vi "Keithley Source Control Panel.vi"(8 "error in (no error)":errorcluster, 11 "Class":refnum<class "Keithley Source.lvclass">) -> (0 "error out":errorcluster, 3 "Keithley Source out":refnum<class "Keithley Source.lvclass">)   [LabVIEW 2015, in "Keithley Source.lvclass"]
uses:
  Keithley Source.lvclass
  Kethley Source Data.ctl
panel:
  in  "Data":T1={"Mode"=enum."up-down sweep", "Start current"=-2e-08, "End current"=2e-08, "Current step"=1e-09, "Compliance"=0.0} {"Compliance" format="%#_4p"; "Current step" format="%#_4p"; "End current" format="%#_4p"; "Start current" format="%#_4p"}
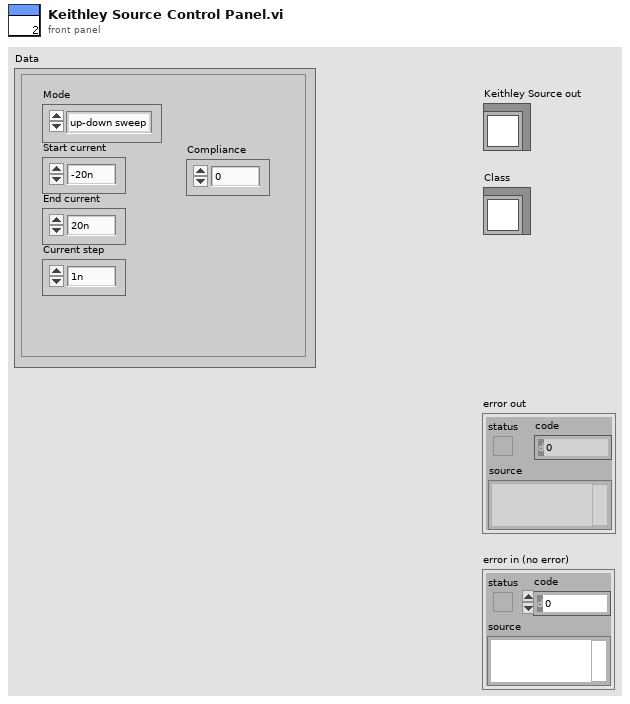
[diagram p1: front panel]
types:
  T1 = typedef "Kethley Source Data.ctl" = cluster{"Mode":enum16{"up-down sweep"}, "Start current":dbl, "End current":dbl, "Current step":dbl, "Compliance":dbl}
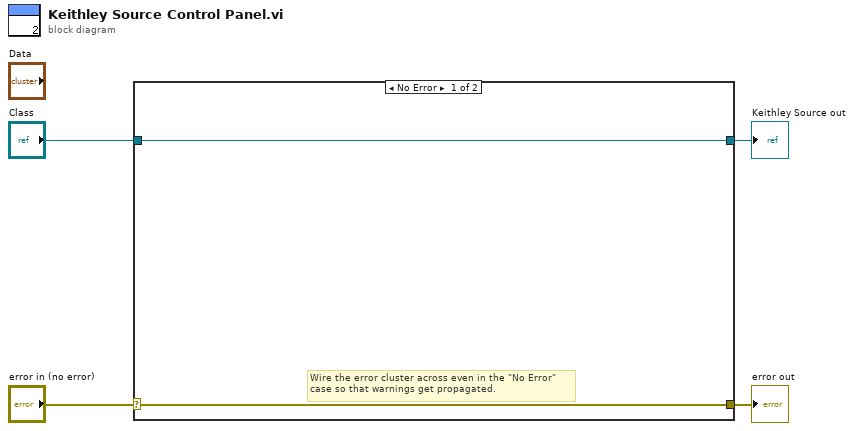
[diagram p0: block diagram]
diagram:
  n1 = case shown="No Error" "error in (no error)" {
    selector: "error in (no error)" -> [w5 w8]
    tunnel: [w5 w8] -> w3
    tunnel: [w6 w7] -> w1
    tunnel: "Class" -> [w6 w7]
    frame No Error {
      # "Wire the error cluster across even in the \"No Error\"\ncase so that warnings get propagated."
    }
    frame Error {
    }
  }
  "error out" <- w3
  "Keithley Source out" <- w1
